vi "Translation2d_GetAngle.vi"(11 "In Translation":T2 {"Y" format="%14.3f"; "X" format="%14.3f"}) -> (3 "Angle_Rotation2d":T1={"VALUE"=0.0, "COS"=1.0, "SIN"=0.0} {"SIN" format="%13.4f"; "COS" format="%13.4f"; "VALUE" format="%13.4f"})   [LabVIEW 2019, in "Trajectory_Library.lvlib"]
doc: "Returns the angle this translation forms with the positive X axis.\n\n\nParameters: \n - IN TRANSLATION2d - This TRANSLATION2 data structure\n\nReturns:\n - Angle -- The angle of the translation (Radians)"
uses:
  Trajectory_Library.lvlib
  TypeDef/TRANSLATION2D.ctl
  TypeDef/ROTATION2D.ctl
  Util_CalcDist.vi
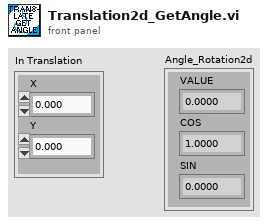
[diagram p1: front panel]
types:
  T1 = typedef "Trajectory_Library.lvlib/ROTATION2D.ctl" = cluster{"VALUE":dbl, "COS":dbl, "SIN":dbl}
  T2 = typedef "Trajectory_Library.lvlib/TRANSLATION2D.ctl" = cluster{"X":dbl, "Y":dbl}
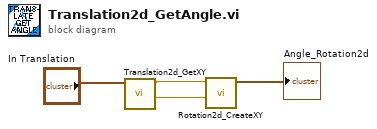
[diagram p0: block diagram]
diagram:
  n1 = call "Translation2d_GetXY.vi"("In Translation"="In Translation") -> ("Y"=w2:dbl, "X"=w3:dbl)  [unwired: 9 in]
  n2 = call "Rotation2d_CreateXY.vi"("Y or sine"=w2, "X or  cosine"=w3) -> ("ROTATION"=→"Angle_Rotation2d":T1)  [unwired: 9 in]
